vi "DS345 tw.vi"(8 "Update":bool, 10 "Cluster":T1={"Osc. Amp. (V)"=0.06, "Osc. Freq. (Hz)"=1000.0} {"Osc. Freq. (Hz)" min=0.001 max=250000.0 step=0.001 format="%.3f"; "Osc. Amp. (V)" min=0.001 max=10.0 step=0.001 format="%.3f"}, 11 "SRS DS345 GPIB address":string="0:19") -> ()   [LabVIEW 2015]
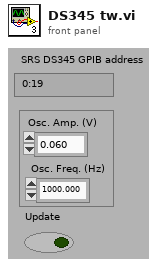
[diagram p1: front panel]
types:
  T1 = cluster{"Osc. Amp. (V)":dbl, "Osc. Freq. (Hz)":dbl}
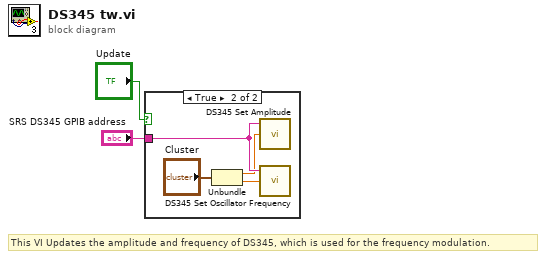
[diagram p0: block diagram]
diagram:
  # "This VI Updates the amplitude and frequency of DS345, which is used for the frequency modulation."
  n1 = case shown="True" "Update" {
    tunnel: "SRS DS345 GPIB address" -> [_ w6]
    frame False {
    }
    frame True {
      n2 = Unbundle("Cluster") -> ("Osc. Amp. (V)"=w3:dbl, "Osc. Freq. (Hz)"=w4:dbl)
      n3 = call "DS345 Set Amplitude.vi"("Oscillator Amplitude (V)"=w3, "GPIB address"=w6) -> ()  [unwired: 1 in, 3 out]
      n4 = call "DS345 Set Oscillator Frequency.vi"("Freq. (Hz)"=w4, "GPIB address"=w6) -> ()  [unwired: 2 in, 2 out]
    }
  }
